vi "UpdateControls.vi"(5 "timeout in ms (1000ms)":i32=1000, 7 "ControlToCommand":map{refnum<vi>, string[]}(c390), 8 "IO Queue":refnum<queue>) -> (0 "timed out?":bool)   [LabVIEW 2020]
uses:
  <vilib>/regexp/Match Regular Expression.xnode
  b4b72fbe-0d65-4e34-aed1-945e0fd32edb.vi
  <vilib>/Utility/Data Type/NI_Data Type.lvlib
  a61e12f5-7996-4f90-b0c7-17f725a99135.vi
  TextControlledInstrumIOQueuePacket.ctl
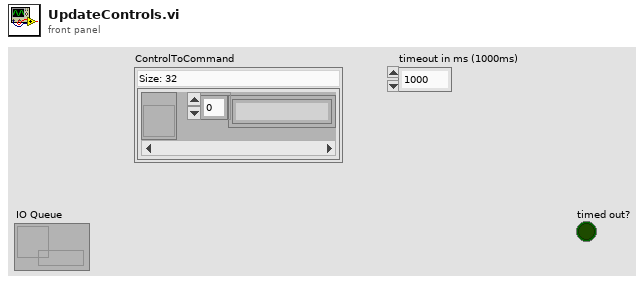
[diagram p1: front panel]
types:
  T1 = typedef "NI_Data Type.lvlib/Data Type.ctl" = enum8{"Invalid Type", "Void", "I8", "I16", "I32", "I64", "U8", "U16", "U32", "U64", "Single Float", "Double Float", "Extended Float", "Single Complex", "Double Complex", "Extended Complex", "Enum U8", "Enum U16", "Enum U32", "Enum U64", "Single Float With Unit", "Double Float With Unit", "Extended Float With Unit", "Single Complex with Unit", "Double Complex with Unit", "Extended Complex with Unit", "Boolean", "String", "Path", "Picture", "Tag", "Array", "Cluster", "Variant", "LV Variant", "Waveform", "Timestamp", "Digital Waveform", "Digital Data", "ExpressData", "Refnum", "External Data", "VI", "Poly VI", "LabVIEW Class Instance", "Fixed Point", "Set Collection", "Map Collection"}
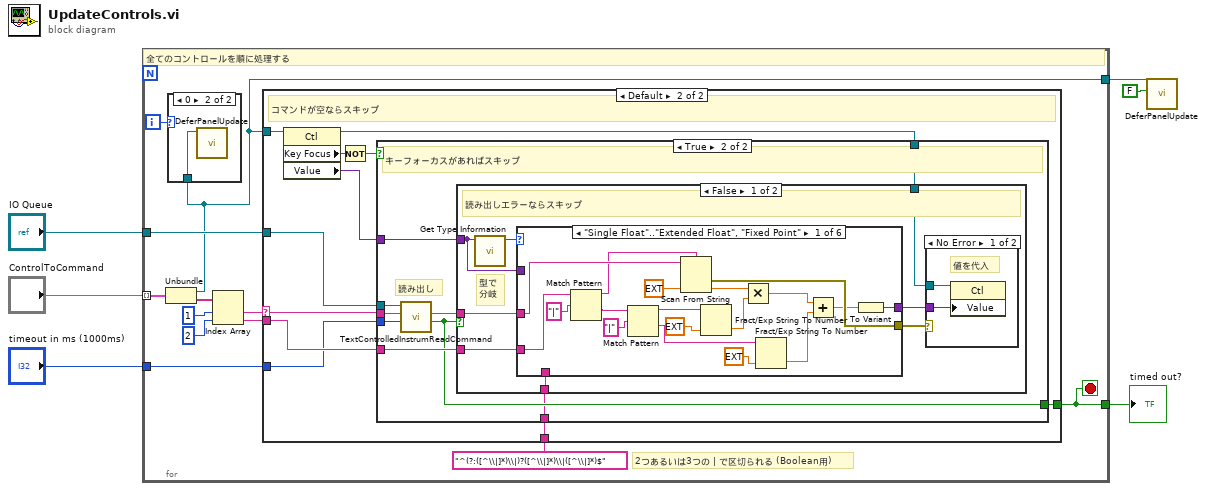
[diagram p0: block diagram]
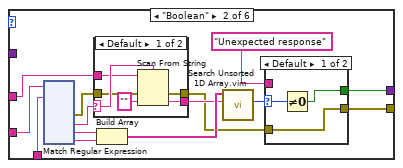
[diagram p6: hidden frame]
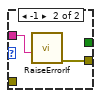
[diagram p7: hidden frame]
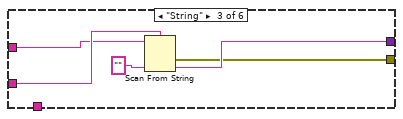
[diagram p9: hidden frame]
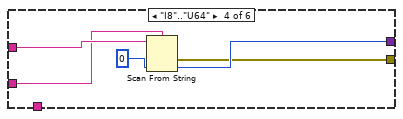
[diagram p10: hidden frame]
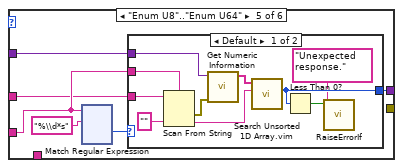
[diagram p11: hidden frame]
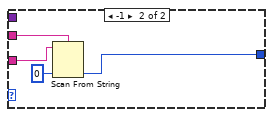
[diagram p12: hidden frame]
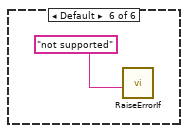
[diagram p13: hidden frame]
diagram:
  n1 = for {
    tunnel: "ControlToCommand" -> [w18] mode=indexing
    tunnel: "timeout in ms (1000ms)" -> [w10]
    tunnel: "IO Queue" -> [w11]
    tunnel: [w9] -> w3
    tunnel: [w7] -> w2
    i -> [w8]
    stop <- w9 stop-if-true
    # "2つあるいは3つの | で区切られる (Boolean用)"
    # "全てのコントロールを順に処理する"
    n2 = Unbundle(w18) -> (w7:refnum<vi>, w12:string[])
    n3 = case shown="0" w8 {
      tunnel: w7 -> [_ w19]
      frame Default {
      }
      frame 0 {
        n4 = call "DeferPanelUpdate.vi"("Control in"=w19) -> ()  [unwired: 8 in, 3 out]
      }
    }
    n5 = Index Array(array=w12, index #1=1 ("index"), index #2=2 ("index")) -> (element #1=w17:string, element #2=w16:string)
    n6 = case shown="Default" w17 {
      selector: w17 -> [_ w21]
      tunnel: w11 -> [_ w30]
      tunnel: [_ w29] -> w9
      tunnel: w7 -> [_ w28]
      tunnel: w16 -> [_ w24]
      tunnel: w10 -> [_ w23]
      tunnel: "^(?:([^\\|]*)\\|)?([^\\|]*)\\|([^\\|]*)$" ("regular expression") -> [_ w20]
      frame "" {
      }
      frame Default {
        # "コマンドが空ならスキップ"
        n7 = property class="Ctl"(reference=w28) -> (reference out=w25:refnum<vi>, "Key Focus"=w26:bool, "Value"=w22:variant)  [unwired: 1 in, 1 out]
        n8 = Not(x=w26) -> (.not. x?=w27:bool)
        n9 = case shown="True" w27 {
          tunnel: w21 -> [_ w34]
          tunnel: w30 -> [_ w36]
          tunnel: w22 -> [_ w39]
          tunnel: [_ w32] -> w29
          tunnel: w25 -> [_ w38]
          tunnel: w24 -> [_ w37]
          tunnel: w23 -> [_ w33]
          tunnel: w20 -> [_ w31]
          frame False {
            # "フォーカスがあるのでスキップ"
          }
          frame True {
            # "読み出し"
            # "キーフォーカスがあればスキップ"
            n10 = call "TextControlledInstrumReadCommand.vi"("timeout in ms (100)"=w33, "Command"=w34, "IO Queue"=w36) -> ("timed out?"=w32:bool, "Received"=w35:string)  [unwired: 6 in, 1 out]
            n11 = case shown="False" w32 {
              tunnel: w39 -> [w40 _]
              tunnel: w38 -> [w46 _]
              tunnel: w37 -> [w44 _]
              tunnel: w35 -> [w42 _]
              tunnel: w31 -> [w41 _]
              frame False {
                # "型で\n分岐"
                # "読み出しエラーならスキップ"
                n12 = call <vilib>:"Get Type Information.vi"("variant"=w40) -> ("type"=w47:T1)  [unwired: 6 in, 4 out]
                n13 = case shown="\"Single Float\"..\"Extended Float\", \"Fixed Point\"" w47 {
                  tunnel: w44 -> [w61 w81 w219 w224 w229 _]
                  tunnel: w42 -> [w67 w78 w217 w225 w228 _]
                  tunnel: [w64 w71 w220 w222 w227 _] -> w45
                  tunnel: w41 -> [_ w80 _ _ _ _]
                  tunnel: [w63 w70 w216 w221 _ _] -> w43
                  tunnel: w40 -> [_ _ _ _ w226 _]
                  frame "Single Float".."Extended Float", "Fixed Point" {
                    n14 = Match Pattern(string=w61, regular expression="|") -> (before substring=w60:string, after substring=w55:string)  [unwired: 1 in, 2 out]
                    n15 = Match Pattern(string=w55, regular expression="|") -> (before substring=w54:string, after substring=w56:string)  [unwired: 1 in, 2 out]
                    n16 = Scan From String(format string=w60, input string=w67, default 1=ext 0.0 ("default value 1")) -> (error out=w63:errorcluster, output 1=w65:ext)  [unwired: 2 in, 2 out]
                    n17 = Fract/Exp String To Number(string=w54, default (0 dbl)=ext 1.0 ("default (0 DBL)")) -> (number=w53:ext)  [unwired: 2 in, 1 out]
                    n18 = Multiply(x=w65, y=w53) -> (x*y=w51:ext)
                    n19 = Fract/Exp String To Number(string=w56, default (0 dbl)=ext 0.0 ("default (0 DBL)")) -> (number=w50:ext)  [unwired: 2 in, 1 out]
                    n20 = Add(x=w51, y=w50) -> (x+y=w52:ext)
                    n21 = To Variant(anything=w52) -> (Variant=w64:variant)
                  }
                  frame "Boolean" {
                    n22 = xnode "Match Regular Expression"("input string"=w81, "regular expression"=w80) -> ("error out"=w69:errorcluster, "submatch 1"=w79:string, "submatch 2"=w77:string, "submatch 3"=w76:string)  [unwired: 4 in, 4 out]
                    n23 = case shown="Default" w79 {
                      selector: w79 -> [w92 _]
                      tunnel: w78 -> [w91 w94]
                      tunnel: [w89 w94] -> w74
                      tunnel: [w88 w93] -> w68
                      tunnel: w69 -> [w87 w93]
                      frame Default {
                        n24 = Scan From String(format string=w92, input string=w91, error in=w87, default 1="" ("submatch 1")) -> (error out=w88:errorcluster, output 1=w89:string)  [unwired: 1 in, 2 out]
                      }
                      frame "" {
                      }
                    }
                    n25 = Build Array(w77, w76) -> (w75:string[])
                    n26 = call "Search Unsorted 1D Array.vim"("element"=w74, "unsorted 1D array"=w75) -> ("index of element"=w73:i32)  [unwired: 9 in]
                    n27 = case shown="Default" w73 {
                      selector: w73 -> [w84 _]
                      tunnel: "Unexpected response" ("submatch 1") -> [_ w86]
                      tunnel: [w83 _] -> w71
                      tunnel: [w82 w85] -> w70
                      tunnel: w68 -> [w82 _]
                      frame Default {
                        n28 = Not Equal To 0?(x=w84) -> (x != 0?=w83:bool)
                      }
                      frame -1 {
                        n29 = call "RaiseErrorIf.vi"("error message"=w86) -> ("error out"=w85:errorcluster)  [unwired: 10 in]
                      }
                    }
                  }
                  frame "String" {
                    n30 = Scan From String(format string=w219, input string=w217, default 1="") -> (error out=w216:errorcluster, output 1=w220:string)  [unwired: 2 in, 2 out]
                  }
                  frame "I8".."U64" {
                    n31 = Scan From String(format string=w224, input string=w225, default 1=i64 0 ("default value 1")) -> (error out=w221:errorcluster, output 1=w222:i64)  [unwired: 2 in, 2 out]
                  }
                  frame "Enum U8".."Enum U64" {
                    n32 = xnode "Match Regular Expression"("input string"=w229, "regular expression"="%\\d*s") -> ("offset past match"=w230:i32)  [unwired: 4 in, 4 out]
                    n33 = case shown="Default" w230 {
                      tunnel: w229 -> [w241 w245]
                      tunnel: w228 -> [w240 w244]
                      tunnel: [w234 w242] -> w227
                      tunnel: w226 -> [w237 _]
                      frame Default {
                        n34 = Scan From String(format string=w241, input string=w240, default 1="") -> (error out=w238:errorcluster, output 1=w235:string)  [unwired: 2 in, 2 out]
                        n35 = call <vilib>:"Get Numeric Information.vi"("error in (no error)"=w238, "variant"=w237) -> ("enum names"=w236:string[])  [unwired: 6 in, 3 out]
                        n36 = call "Search Unsorted 1D Array.vim"("element"=w235, "unsorted 1D array"=w236) -> ("index of element"=w234:i32)  [unwired: 9 in]
                        n37 = Less Than 0?(x=w234) -> (x < 0?=w233:bool)
                        n38 = call "RaiseErrorIf.vi"("error message"="Unexpected response.", "error? (true)"=w233) -> ()  [unwired: 9 in, 1 out]
                      }
                      frame -1 {
                        n39 = Scan From String(format string=w245, input string=w244, default 1=u32 0 ("default value 1")) -> (output 1=w242:u32)  [unwired: 2 in, 3 out]
                      }
                    }
                  }
                  frame Default {
                    n40 = call "RaiseErrorIf.vi"("error message"="not supported" ("error source (\" \")")) -> ()  [unwired: 10 in, 1 out]
                  }
                }
                n41 = case shown="No Error" w43 {
                  tunnel: w46 -> [w49 _]
                  tunnel: w45 -> [w48 _]
                  frame No Error {
                    # "値を代入"
                    n42 = property class="Ctl"(reference=w49, "Value"=w48) -> ()  [unwired: 1 in, 2 out]
                  }
                  frame Error {
                  }
                }
              }
              frame True {
              }
            }
          }
        }
      }
    }
  }
  "timed out?" <- w3
  n43 = call "DeferPanelUpdate.vi"("Defer Panel Updates (T)"=FALSE, "Control in"=w2) -> ()  [unwired: 7 in, 3 out]
